vi "Vertical Panel.vi"() -> ()   [LabVIEW 2013, in "PanelDataNode.lvclass"]
uses:
  PanelDataNode.lvclass
  PanelObject/PanelObject.lvclass
  Split Mode.ctl
  PanelLinkNode/PanelLinkNode.lvclass
panel:
  in  "Node*":refnum<data-value>
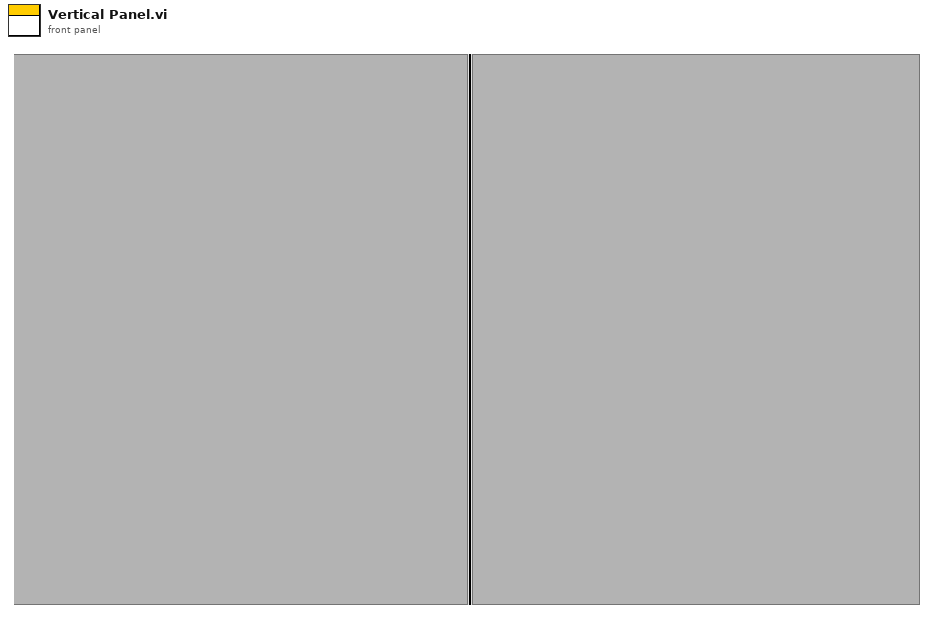
[diagram p1: front panel]
types:
  T1 = typedef "PanelDataNode.lvclass/Split Mode.ctl" = enum16{"Horizontal(up)", "Vertical(left)", "Horizontal(down)", "Vertical(right)"}
  T2 = cluster{"ChildNode*":refnum<data-value>, "Split Mode":T1}
  T3 = cluster{"ChildNode*":refnum<data-value>, "VI*":refnum<vi>}
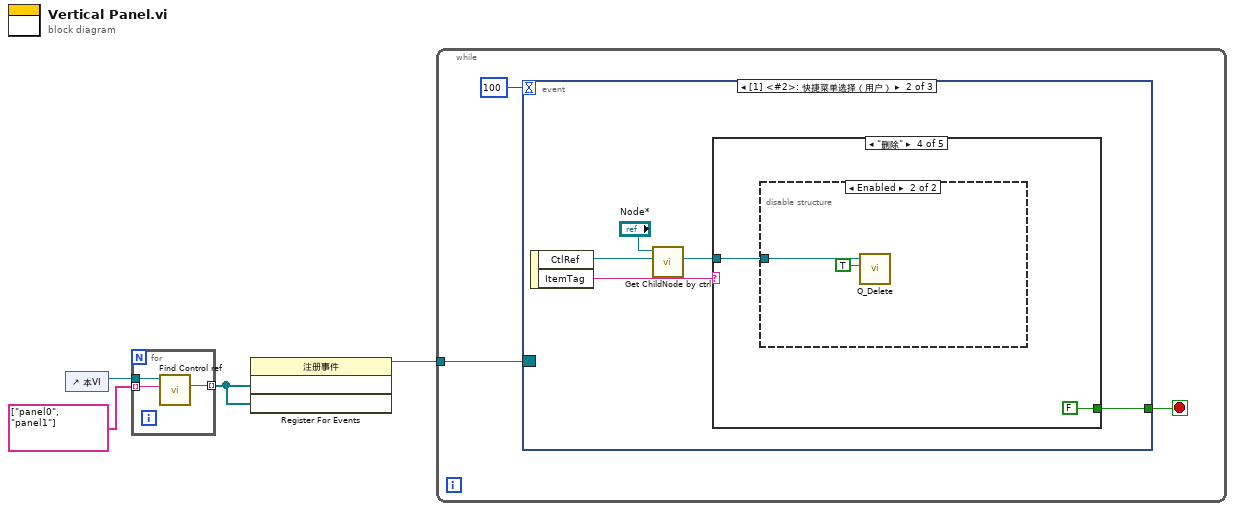
[diagram p0: block diagram]
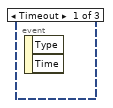
[diagram p2: hidden frame]
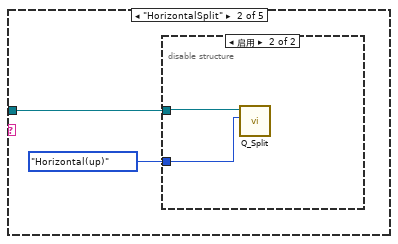
[diagram p4: hidden frame]
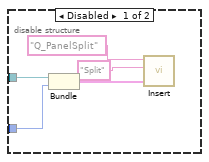
[diagram p5: hidden frame]
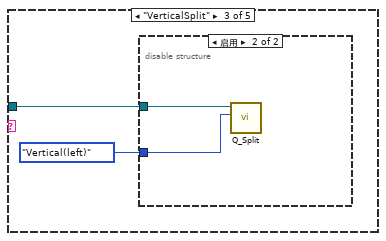
[diagram p6: hidden frame]
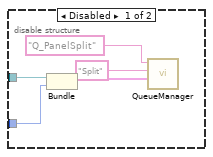
[diagram p7: hidden frame]
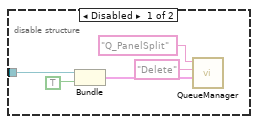
[diagram p8: hidden frame]
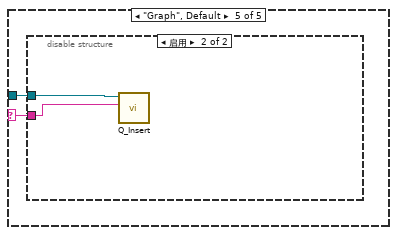
[diagram p9: hidden frame]
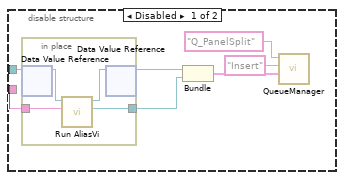
[diagram p10: hidden frame]
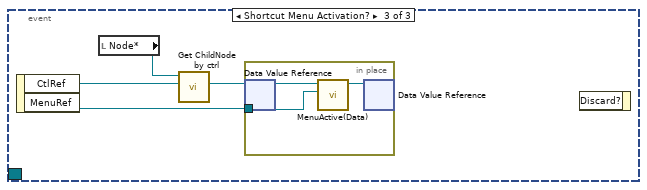
[diagram p11: hidden frame]
diagram:
  n1 = control-ref of="本VI"() -> (w4:refnum<vi>)
  n2 = for {
    tunnel: w4 -> [w7]
    tunnel: string[] ["panel0", "panel1"] -> [w6] mode=indexing
    tunnel: [w5] -> w1 mode=indexing
    n3 = call "Find Control ref.vi"("control name"=w6, "panelvi*"=w7) -> ("ctrl*"=w5:refnum<vi>)  [unwired: 7 in, 2 out]
  }
  n4 = register-events(w1, w1) -> (reference out=w2:refnum<event-registration>)  [unwired: 2 in, 1 out]
  n5 = while {
    tunnel: w2 -> [w9]
    stop <- w8 stop-if-true
    n6 = event shown="[1] <#2>: 快捷菜单选择（用户）" {
      selector: w9 -> [_ _ _]
      dyn-events: _ -> [_ _ _]
      timeout: 100 -> [_ _ _]
      tunnel: [_ w11 _] -> w8
      event Timeout {
        n7 = event-data() -> ()  [unwired: 1 in, 2 out]
      }
      event Shortcut Menu Selection (User) {
        n8 = event-data() -> ("CtlRef"=w15:refnum<vi>, "ItemTag"=w12:string)  [unwired: 1 in]
        n9 = call "Get ChildNode by ctrl.vi"("ctr*"=w15, "Node*"="Node*") -> ("ChildNode*"=w13:refnum<data-value>)  [unwired: 8 in, 1 out]
        n10 = case shown="\"删除\"" w12 {
          selector: w12 -> [_ _ _ _ w44]
          tunnel: w13 -> [_ w17 w25 w34 w43]
          tunnel: [_ _ _ FALSE _] -> w11
          frame "假" {
          }
          frame "HorizontalSplit" {
            n11 = disable-structure shown="启用" {
              disable-tunnel: w17 -> [w22 w24]
              disable-tunnel: Split_Mode."Horizontal(up)" ("Split Mode") -> [w21 w23]
              frame Disabled {
                n12 = Bundle("ChildNode*"=w22, "Split Mode"=w21) -> (w20:T2)  [unwired: 1 in]
                n13 = call "Insert.vi"("Data"=w20, "Event"="Split", "QueueName"="Q_PanelSplit") -> ()  [unwired: 7 in, 2 out]
              }
              frame Enabled {
                n14 = call "Q_Split.vi"("Split Mode"=w23, "ChildNode*"=w24) -> ()  [unwired: 9 in, 1 out]
              }
            }
          }
          frame "VerticalSplit" {
            n15 = disable-structure shown="启用" {
              disable-tunnel: Split_Mode."Vertical(left)" ("Split Mode") -> [w31 w33]
              disable-tunnel: w25 -> [w30 w32]
              frame Disabled {
                n16 = Bundle("ChildNode*"=w30, "Split Mode"=w31) -> (w27:T2)  [unwired: 1 in]
                n17 = call-poly "QueueManager.vi"("Data"=w27, "Event"="Split", "QueueName"="Q_PanelSplit") -> ()  [unwired: 7 in, 2 out]
              }
              frame Enabled {
                n18 = call "Q_Split.vi"("Split Mode"=w33, "ChildNode*"=w32) -> ()  [unwired: 9 in, 1 out]
              }
            }
          }
          frame "删除" {
            n19 = disable-structure shown="Enabled" {
              disable-tunnel: w34 -> [w40 w42]
              frame Disabled {
                n20 = Bundle("ChildNode*"=w40, TRUE) -> (w39:cluster{"ChildNode*":refnum<data-value>, bool})  [unwired: 1 in]
                n21 = call-poly "QueueManager.vi"("Data"=w39, "Event"="Delete", "QueueName"="Q_PanelSplit") -> ()  [unwired: 7 in, 2 out]
              }
              frame Enabled {
                n22 = call "Q_Delete.vi"("CloseVI?(T)"=TRUE, "ChildNode*"=w42) -> ()  [unwired: 9 in, 1 out]
              }
            }
          }
          frame "Graph", Default {
            n23 = disable-structure shown="启用" {
              disable-tunnel: w44 -> [w48 w56]
              disable-tunnel: w43 -> [w47 w57]
              frame Disabled {
                n24 = in-place {
                  in-place-border: w48 -> [w55]
                  in-place-border: [w52] -> w45
                  n25 = in-place-dvr #1(w47) -> (w54:refnum<class "PanelDataNode.lvclass">)  [unwired: 1 out]
                  n26 = call-dynamic "Run AliasVi.vi"("Vi Alias"=w55, "PanelDataNode 输入"=w54) -> ("VI*"=w52:refnum<vi>, "PanelDataNode 输出"=w53:refnum<class "PanelDataNode.lvclass">)  [unwired: 7 in, 1 out]
                  n27 = in-place-dvr #1(w53) -> (w46:refnum<data-value>)  [unwired: 1 out]
                }
                n28 = Bundle("ChildNode*"=w46, "VI*"=w45) -> (w51:T3)  [unwired: 1 in]
                n29 = call-poly "QueueManager.vi"("Data"=w51, "Event"="Insert", "QueueName"="Q_PanelSplit") -> ()  [unwired: 7 in, 2 out]
              }
              frame Enabled {
                n30 = call "Q_Insert.vi"("Vi Alias"=w56, "ChildNode*"=w57) -> ()  [unwired: 9 in, 1 out]
              }
            }
          }
        }
      }
      event Shortcut Menu Activation? {
        n31 = event-data() -> ("CtlRef"=w61:refnum<vi>, "MenuRef"=w58:refnum<k9>)  [unwired: 1 in]
        n32 = local read "Node*"() -> (w60:refnum<data-value>)
        n33 = call "Get ChildNode by ctrl.vi"("ctr*"=w61, "Node*"=w60) -> ("ChildNode*"=w59:refnum<data-value>)  [unwired: 8 in, 1 out]
        n34 = in-place {
          in-place-border: w58 -> [w63]
          n35 = in-place-dvr #2(w59) -> (w64:refnum<class "PanelDataNode.lvclass">)  [unwired: 1 out]
          n36 = call-dynamic "MenuActive(Data).vi"("菜单引用"=w63, "PanelDataNode 输入"=w64) -> ("PanelDataNode 输出"=w62:refnum<class "PanelDataNode.lvclass">)  [unwired: 7 in, 2 out]
          n37 = in-place-dvr #2(w62) -> ()  [unwired: 2 out]
        }
        n38 = event-data() -> ()  [unwired: 2 in, 1 out]
      }
    }
  }
